vi "List Feeds Containing Package.vi"(8 "error in":errorcluster, 11 "package name":string) -> (0 "error out":errorcluster, 2 "feeds":T1[](array[typedef]))   [LabVIEW 2014, in "NIPM_API.lvlib"]
doc: "Lists all the registered feeds that contain the specified package.\n\nINPUT(s)\n<B>Package name</B>: Specify the package name. This VI returns Error 5011 if Package Name is an empty string.\n\nOUTPUT(s)\n<B>Feeds</B>: Lists all the registered feeds that contain the specified package. If no registered feeds contain the specified package, then this output returns an empty array."
uses:
  NIPM_API.lvlib
  _support/feed.ctl
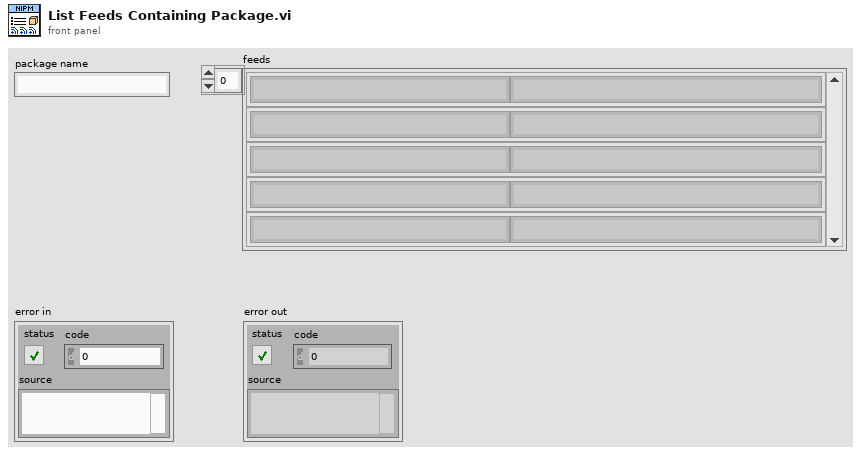
[diagram p1: front panel]
types:
  T1 = typedef "NIPM_API.lvlib/feed.ctl" = cluster{"Name":string, "URI":string}
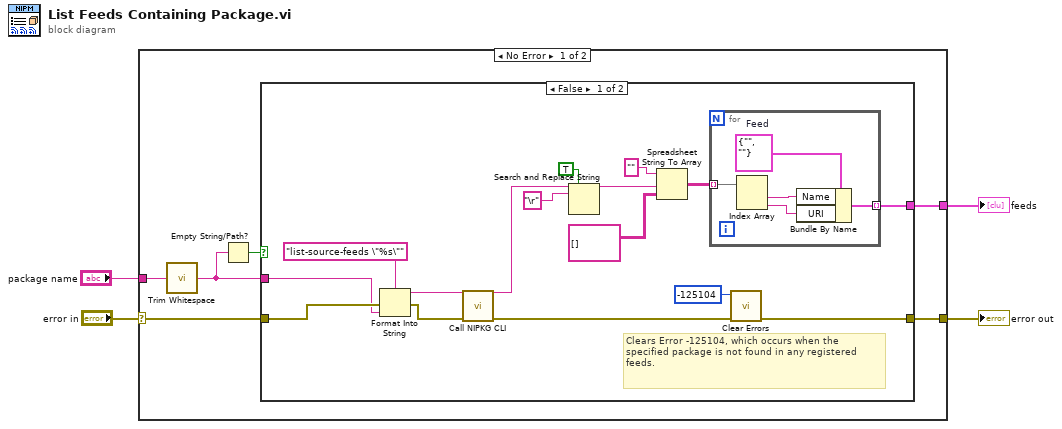
[diagram p0: block diagram]
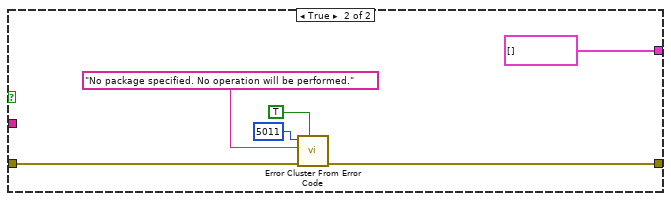
[diagram p2: hidden frame]
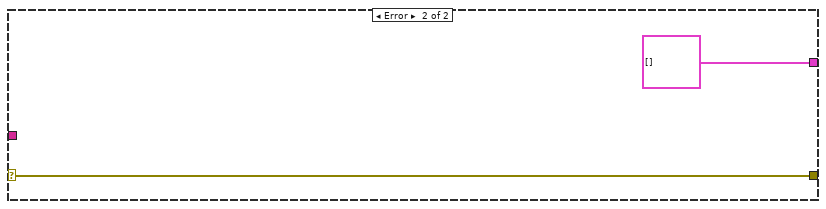
[diagram p3: hidden frame]
diagram:
  n1 = case shown="No Error" "error in" {
    selector: "error in" -> [w8 w39]
    tunnel: [w10 w39] -> w3
    tunnel: [w9 T1[] []] -> w2
    tunnel: "package name" -> [w7 _]
    frame No Error {
      n2 = call <vilib>:"Trim Whitespace.vi"("string"=w7) -> ("trimmed string"=w6:string)  [unwired: 1 in]
      n3 = Empty String/Path?(string/path=w6) -> (empty?=w5:bool)
      n4 = case shown="False" w5 {
        tunnel: [w12 w33] -> w10
        tunnel: [w19 T1[] []] -> w9
        tunnel: w8 -> [w16 w34]
        tunnel: w6 -> [w14 _]
        frame False {
          # "Clears Error -125104, which occurs when the specified package is not found in any registered feeds."
          n5 = Format Into String(format string="list-source-feeds \"%s\"", error in=w16, w14) -> (resulting string=w17:string, error out=w15:errorcluster)  [unwired: 1 in]
          n6 = call "Call NIPKG CLI.vi"("error in (no error)"=w15, "command"=w17) -> ("error out"=w13:errorcluster, "command line standard output"=w21:string)  [unwired: 8 in]
          n7 = Search and Replace String(replace all?=TRUE ("replace all? (F)"), input string=w21, search string="\r") -> (result string=w24:string)  [unwired: 5 in, 3 out]
          n8 = Spreadsheet String To Array(format string="", spreadsheet string=w24, array type (2D Dbl)=string[][] []) -> (array=w20:string[][])  [unwired: 1 in]
          n9 = for {
            tunnel: w20 -> [w31] mode=indexing
            tunnel: [w27] -> w19 mode=indexing
            w30 = T1 {"Name"="", "URI"=""}  # Feed
            n10 = Index Array(array=w31) -> (element #1=w29:string, element #2=w28:string)  [unwired: 2 in]
            n11 = Bundle By Name(cluster=w30, "Name"=w29, "URI"=w28) -> (w27:T1)
          }
          n12 = call <vilib>:"Clear Errors.vi"("error in (no error)"=w13, "specific error code to clear (0: all)"=-125104) -> ("error out"=w12:errorcluster)  [unwired: 4 in, 1 out]
        }
        frame True {
          n13 = call <vilib>:"Error Cluster From Error Code.vi"("show call chain? (False)"=TRUE, "error in (no error)"=w34, "error message (\"\")"="No package specified. No operation will be performed.", "error code (0)"=5011) -> ("error out"=w33:errorcluster)  [unwired: 5 in]
        }
      }
    }
    frame Error {
    }
  }
  "error out" <- w3
  "feeds" <- w2
